vi "osc_int.vi"(0 "VISA resource name":refnum<visa-resource-name>, 1 "Serial Configuration":T1={"Baud Rate"=9600, "Parity"=0, "Stop Bits"=10, "Flow Control"=2} {"Flow Control" items=["None", "XON/XOFF", "RTS/CTS", "XON/XOFF & RTS/CTS", "DTR/DSR", "XON/XOFF & DTR/DSR"]; "Stop Bits" items=["1.0"=10, "1.5"=15, "2.0"=20]; "Parity" items=["None", "Odd", "Even", "Mark", "Space"]; "Baud Rate" items=["300"=300, "600"=600, "1200"=1200, "2400"=2400, "4800"=4800, "9600"=9600, "19200"=19200]}, 2 "ID Query? (T: Yes)":bool=TRUE, 3 "error in (no error)":errorcluster) -> (7 "VISA resource name out":refnum<visa-resource-name>, 10 "error out":errorcluster)   [LabVIEW 2013]
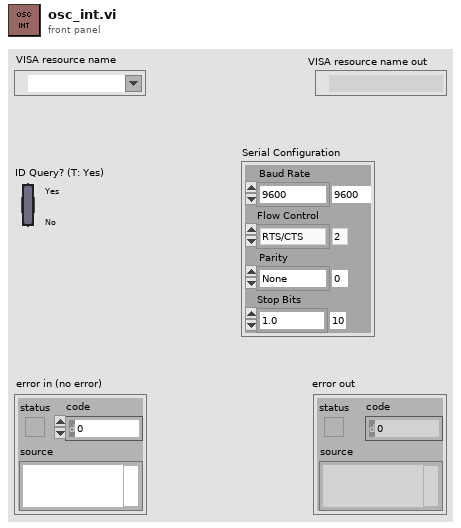
[diagram p1: front panel]
types:
  T1 = cluster{"Baud Rate":u32, "Parity":u16, "Stop Bits":u16, "Flow Control":u16}
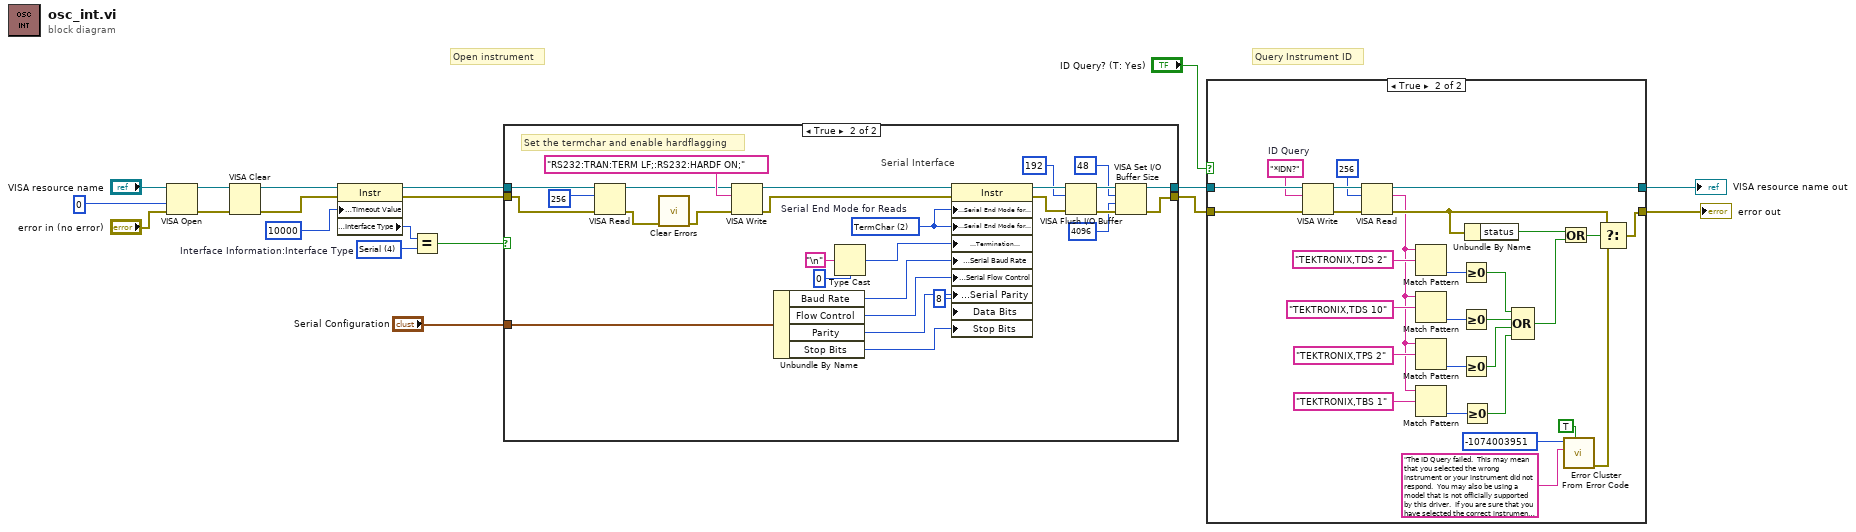
[diagram p0: block diagram]
diagram:
  w9 = u16 4 items=["GPIB"=1, "VXI"=2, "GPIB-VXI"=3, "Serial"=4, "PXI"=5, "TCPIP"=6, "USB"=7]  # Interface Information:Interface Type
  # "Query Instrument ID"
  # "Open instrument"
  n1 = VISA Open(access mode=u32 0, error in (no error)="error in (no error)", VISA resource name="VISA resource name") -> (VISA resource name=w7:refnum<visa-resource-name>, error out=w6:errorcluster)  [unwired: 2 in]
  n2 = VISA Clear(VISA resource name=w7, error in (no error)=w6) -> (VISA resource name out=w5:refnum<visa-resource-name>, error out=w4:errorcluster)
  n3 = property class="Instr"(reference=w5, error in=w4, "General Settings:Timeout Value"=u32 10000) -> (reference out=w12:refnum<visa-resource-name>, error out=w11:errorcluster, "Interface Information:Interface Type"=w16:u16)
  n4 = Equal?(x=w16, y=w9) -> (x = y?=w10:bool)
  n5 = case shown="True" w10 {
    tunnel: [w20 w48] -> w14
    tunnel: [w21 w45] -> w13
    tunnel: w12 -> [w20 w27]
    tunnel: w11 -> [w21 w26]
    tunnel: "Serial Configuration" -> [_ w22]
    frame False {
      # "GPIB Interface"
    }
    frame True {
      w38 = u16 2 items=["None", "LastBit", "TermChar"]  # Serial End Mode for Reads
      # "Set the termchar and enable hardflagging"
      # "Serial Interface"
      n6 = VISA Read(VISA resource name=w27, byte count=u32 256, error in (no error)=w26) -> (VISA resource name out=w25:refnum<visa-resource-name>, error out=w24:errorcluster)  [unwired: 2 out]
      n7 = call <vilib>:"Clear Errors.vi"("error in (no error)"=w24) -> ("error out"=w23:errorcluster)  [unwired: 6 in]
      n8 = VISA Write(VISA resource name=w25, write buffer="RS232:TRAN:TERM LF;:RS232:HARDF ON;", error in (no error)=w23) -> (VISA resource name out=w33:refnum<visa-resource-name>, error out=w32:errorcluster)  [unwired: 1 out]
      n9 = Unbundle By Name(w22) -> ("Baud Rate"=w36:u32, "Flow Control"=w34:u16, "Parity"=w35:u16, "Stop Bits"=w30:u16)
      n10 = Type Cast(type=u8 0, x="\n" ("Line Feed Constant")) -> (*(type *) &x=w37:u8)
      n11 = property class="Instr"(reference=w33, error in=w32, "Serial Settings:Serial End Mode for Reads"=w38, "Serial Settings:Serial End Mode for Writes"=w38, "Message Based Settings:Termination Character"=w37, "Serial Settings:Serial Baud Rate"=w36, "Serial Settings:Serial Flow Control"=w34, "Serial Settings:Serial Parity"=w35, "Data Bits"=u16 8 ("Serial Settings:Serial Data Bits"), "Stop Bits"=w30) -> (reference out=w44:refnum<visa-resource-name>, error out=w47:errorcluster)
      n12 = VISA Flush I/O Buffer(VISA resource name=w44, mask (16)=u16 192, error in (no error)=w47) -> (VISA resource name out=w49:refnum<visa-resource-name>, error out=w46:errorcluster)
      n13 = VISA Set I/O Buffer Size(VISA resource name=w49, mask (16)=u16 48, size (4096)=u32 4096 ("size (0)"), error in (no error)=w46) -> (VISA resource name out=w48:refnum<visa-resource-name>, error out=w45:errorcluster)
    }
  }
  n14 = case shown="True" "ID Query? (T: Yes)" {
    tunnel: [w50 w80] -> w1
    tunnel: [w51 w77] -> w2
    tunnel: w14 -> [w51 w78]
    tunnel: w13 -> [w50 w79]
    frame False {
    }
    frame True {
      w72 = "*IDN?"  # ID Query
      n15 = VISA Write(VISA resource name=w78, write buffer=w72, error in (no error)=w79) -> (VISA resource name out=w76:refnum<visa-resource-name>, error out=w75:errorcluster)  [unwired: 1 out]
      n16 = VISA Read(VISA resource name=w76, byte count=u32 256, error in (no error)=w75) -> (VISA resource name out=w77:refnum<visa-resource-name>, read buffer=w55:string, error out=w66:errorcluster)  [unwired: 1 out]
      n17 = Match Pattern(string=w55, regular expression="TEKTRONIX,TDS 2") -> (offset past match=w65:i32)  [unwired: 1 in, 3 out]
      n18 = Match Pattern(string=w55, regular expression="TEKTRONIX,TDS 10") -> (offset past match=w64:i32)  [unwired: 1 in, 3 out]
      n19 = Match Pattern(string=w55, regular expression="TEKTRONIX,TPS 2") -> (offset past match=w58:i32)  [unwired: 1 in, 3 out]
      n20 = Match Pattern(string=w55, regular expression="TEKTRONIX,TBS 1") -> (offset past match=w53:i32)  [unwired: 1 in, 3 out]
      n21 = Greater Or Equal To 0?(x=w65) -> (x >= 0?=w63:bool)
      n22 = Greater Or Equal To 0?(x=w64) -> (x >= 0?=w62:bool)
      n23 = Greater Or Equal To 0?(x=w58) -> (x >= 0?=w57:bool)
      n24 = Greater Or Equal To 0?(x=w53) -> (x >= 0?=w52:bool)
      n25 = Unbundle By Name(w66) -> ("status"=w56:bool)
      n26 = Compound Arithmetic op=OR(w63, w62, w57, w52) -> (w60:bool)
      n27 = Or(x=w56, y=w60) -> (x .or. y?=w61:bool)
      n28 = call <vilib>:"Error Cluster From Error Code.vi"("show call chain? (False)"=TRUE, "error message (\"\")"="The ID Query failed.  This may mean that you selected the wrong instrument or your instrument did not respond.  You may also be using a model that is not officially supported by this driver.  If you are sure that you have selected the correct instrument and it is responding, try disabling the ID Query." ("Source (VI Name)"), "error code (0)"=-1074003951 ("Code")) -> ("error out"=w71:errorcluster)  [unwired: 6 in]
      n29 = Select(t=w66, s=w61, f=w71) -> (s? t:f=w80:errorcluster)
    }
  }
  "VISA resource name out" <- w2
  "error out" <- w1
